vi "Read Lockin.DAQ.vi"(8 "error in (no error)":errorcluster, 11 "Instrument.Lockin in":refnum<class "Instrument.Lockin.lvclass">) -> (0 "error out":errorcluster, 2 "Instrument.DAQ.lvclass":refnum<class "Instrument.DAQ.lvclass">, 3 "Instrument.Lockin out":refnum<class "Instrument.Lockin.lvclass">)   [LabVIEW 2019, in "Instrument.Lockin.lvclass"]
uses:
  Instrument.Lockin.lvclass
  Instrument.DAQ/Instrument.DAQ.lvclass
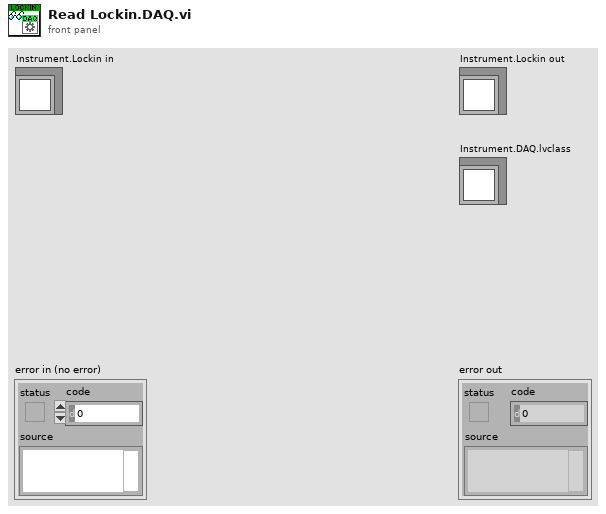
[diagram p1: front panel]
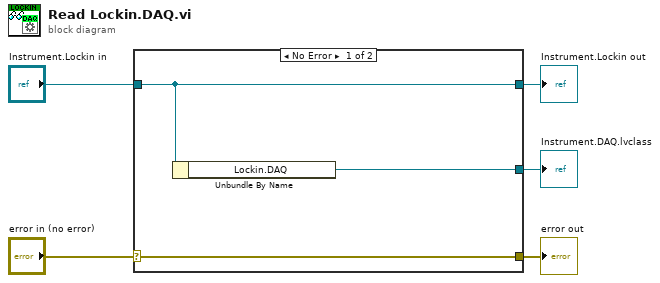
[diagram p0: block diagram]
diagram:
  n1 = case shown="No Error" "error in (no error)" {
    selector: "error in (no error)" -> [w8 w9]
    tunnel: [w8 w9] -> w4
    tunnel: [w7 w10] -> w2
    tunnel: "Instrument.Lockin in" -> [w7 w10]
    tunnel: [w6 _] -> w1
    frame No Error {
      n2 = Unbundle By Name(w7) -> ("Lockin.DAQ"=w6:refnum<class "Instrument.DAQ.lvclass">)
    }
    frame Error {
    }
  }
  "error out" <- w4
  "Instrument.Lockin out" <- w2
  "Instrument.DAQ.lvclass" <- w1
